vi "CRYData View Legend Plot OnOff.vi"(8 "TotalPlot":u32, 9 "Button Info":u16, 10 "Mouse Point":T1, 11 "MCListbox Ref In":refnum<vi>) -> (1 "Active Row":i32, 2 "Visible?":bool, 3 "Click State":bool)   [LabVIEW 2013]
uses:
  <vilib>/Utility/miscctls.llb/LVPositionTypeDef.ctl
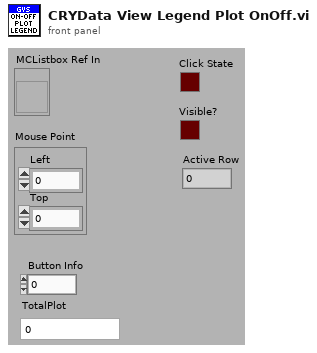
[diagram p1: front panel]
types:
  T1 = typedef "LVPositionTypeDef.ctl" = cluster{"Left":i32, "Top":i32}
  T2 = typedef "LVRowAndColumnTypeDef.ctl" = cluster{"Row":i32, "Column":i32}
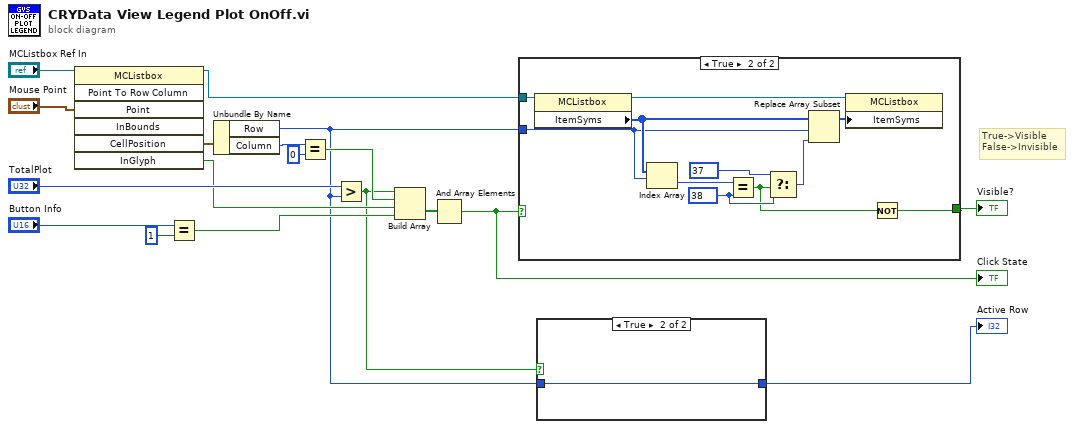
[diagram p0: block diagram]
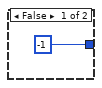
[diagram p2: hidden frame]
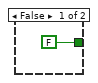
[diagram p3: hidden frame]
diagram:
  # "True->Visible\nFalse->Invisible"
  n1 = invoke on="Invoke Node" class="MCListbox" method="Point To Row Column"(reference="MCListbox Ref In", "Point"="Mouse Point") -> (reference out=w1:refnum<vi>, "CellPosition"=w18:T2, "InGlyph"=w10:bool)  [unwired: 5 in, 4 out]
  n2 = Equal?(x="Button Info", y=u16 1) -> (x = y?=w6:bool)
  n3 = Unbundle By Name(w18) -> ("Row"=w3:i32, "Column"=w9:i32)
  n4 = Equal?(x=w9, y=0) -> (x = y?=w5:bool)
  n5 = Greater?(x="TotalPlot", y=w3) -> (0:w4:bool)
  n6 = Build Array(w4, w5, w10, w6) -> (w16:bool[])
  n7 = And Array Elements(Boolean array=w16) -> (logical AND=w14:bool)
  "Click State" <- w14
  n8 = case shown="True" w14 {
    tunnel: w3 -> [_ w20]
    tunnel: w1 -> [_ w23]
    tunnel: [FALSE w21] -> w15
    frame False {
    }
    frame True {
      w29 = 38
      n9 = property on="Property Node" class="MCListbox"(reference=w23) -> (reference out=w22:refnum<vi>, "ItemSyms"=w27:i32[])  [unwired: 1 in, 1 out]
      n10 = Index Array(array=w27, index=w20) -> (element=w26:i32)
      n11 = Equal?(x=w26, y=w29) -> (x = y?=w24:bool)
      n12 = Select(t=37, s=w24, f=w29) -> (s? t:f=w28:i32)
      n13 = Replace Array Subset(array=w27, new element=w28, index=w20) -> (w30:i32[])
      n14 = property on="Property Node" class="MCListbox"(reference=w22, "ItemSyms"=w30) -> ()  [unwired: 1 in, 2 out]
      n15 = Not(x=w24) -> (.not. x?=w21:bool)
    }
  }
  "Visible?" <- w15
  n16 = case shown="True" w4 {
    tunnel: w3 -> [_ w32]
    tunnel: [-1 ("Row") w32] -> w2
    frame False {
    }
    frame True {
    }
  }
  "Active Row" <- w2
